vi "Read configuration.vi"(8 "error in":errorcluster, 11 "Increment editor node in":refnum<class "Increment editor node.lvclass">) -> (0 "error out":errorcluster, 2 "configuration":refnum<class "NISE_CEF_serializable configuration.lvclass">, 3 "Increment editor node out":refnum<class "Increment editor node.lvclass">)   [LabVIEW 2015, in "Increment editor node.lvclass"]
uses:
  Increment editor node.lvclass
  <vilib>/NI/Configuration Framework/serializable configuration/NISE_CEF_serializable configuration.lvclass
  Increment editor node.lvclass/Increment editor node.ctl
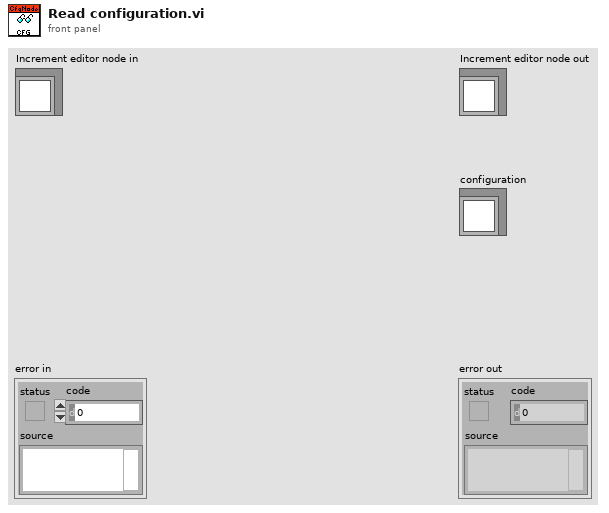
[diagram p1: front panel]
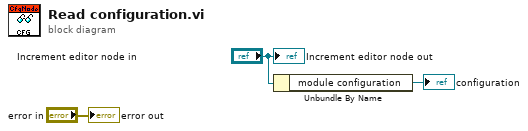
[diagram p0: block diagram]
diagram:
  n1 = Unbundle By Name("Increment editor node in") -> ("module configuration"=→"configuration":refnum<class "Increment configuration.lvclass">)
  "error out" <- "error in"
  "Increment editor node out" <- "Increment editor node in"
